vi "[niDMM] Close All.vi"() -> ()   [LabVIEW 2021]
panel:
  in  "Stop":bool
  in  "Close All session":bool
  out "Instrument Descriptor":refnum<k15>
  out "DropDownList[]":string[](array[string])
  # "NI DMM  Sessions"
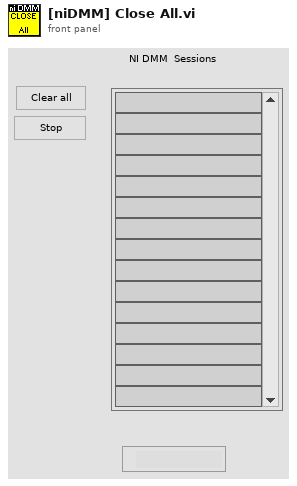
[diagram p1: front panel]
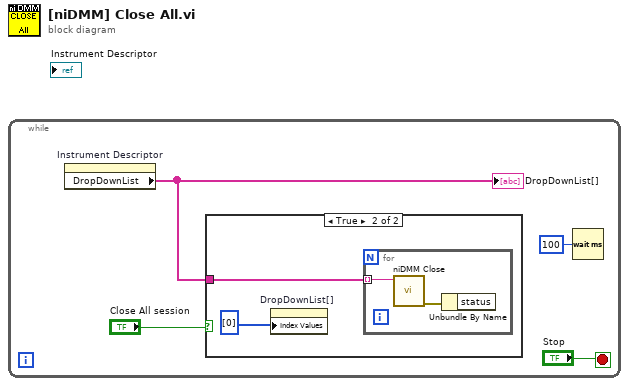
[diagram p0: block diagram]
diagram:
  n1 = while {
    stop <- "Stop" stop-if-true
    n2 = property on="Instrument Descriptor" class="IVIName"() -> ("DropDownList"=w2:string[])  [unwired: 2 in, 2 out]
    "DropDownList[]" <- w2
    n3 = case shown="True" "Close All session" {
      tunnel: w2 -> [_ w6]
      frame False {
      }
      frame True {
        n4 = property on="DropDownList[]" class="Arr (strict)"("Index Values"=u32[] [0]) -> ()  [unwired: 2 in, 2 out]
        n5 = for {
          tunnel: w6 -> [w8] mode=indexing
          n6 = call <instrlib>:"niDMM Close.vi"("instrument handle"=w8) -> ("error out"=w7:errorcluster)  [unwired: 10 in]
          n7 = Unbundle By Name(w7) -> ()  [unwired: 1 out]
        }
      }
    }
    n8 = Wait (ms)(milliseconds to wait=u32 100) -> ()  [unwired: 1 out]
  }
